vi "FTW-HTTPClient-AddHeaders.vi"(0 "HTTP Client":refnum<class "FTW-HTTPClient.lvclass">, 5 "Headers":T1[](array[typedef]), 11 "error in":errorcluster) -> (4 "HTTP Client out":refnum<class "FTW-HTTPClient.lvclass">, 15 "error out":errorcluster)   [LabVIEW 2012, in "FTW-HTTPClient.lvclass"]
uses:
  FTW-HTTPClient.lvclass
  Collection/FTW-Collection-KeyValuePair.ctl
  FTW-HTTPClient.lvclass/FTW-HTTPClient.ctl
panel:
  # "Inputs"
  # "Outputs"
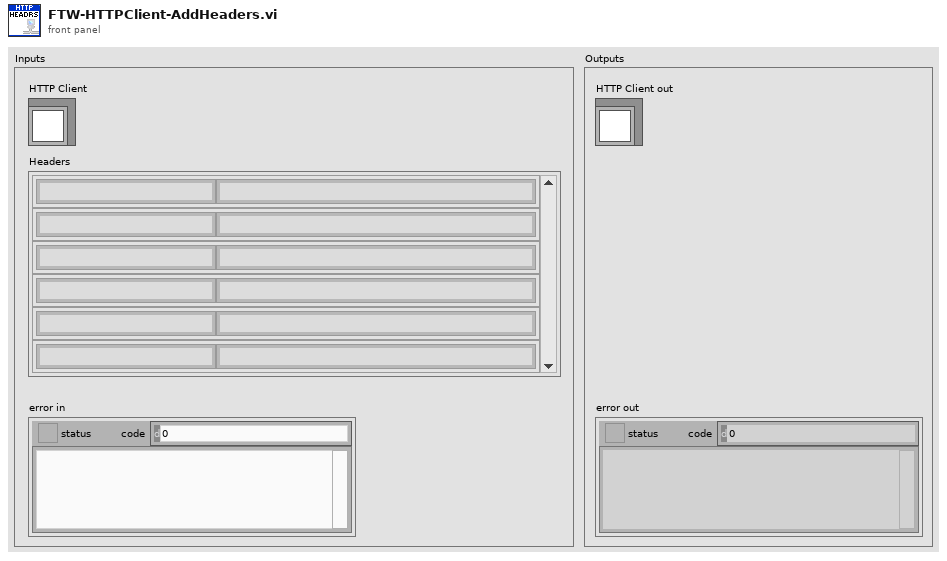
[diagram p1: front panel]
types:
  T1 = typedef "FTW-Collection-KeyValuePair.ctl" = cluster{"Key":string, "Value":string}
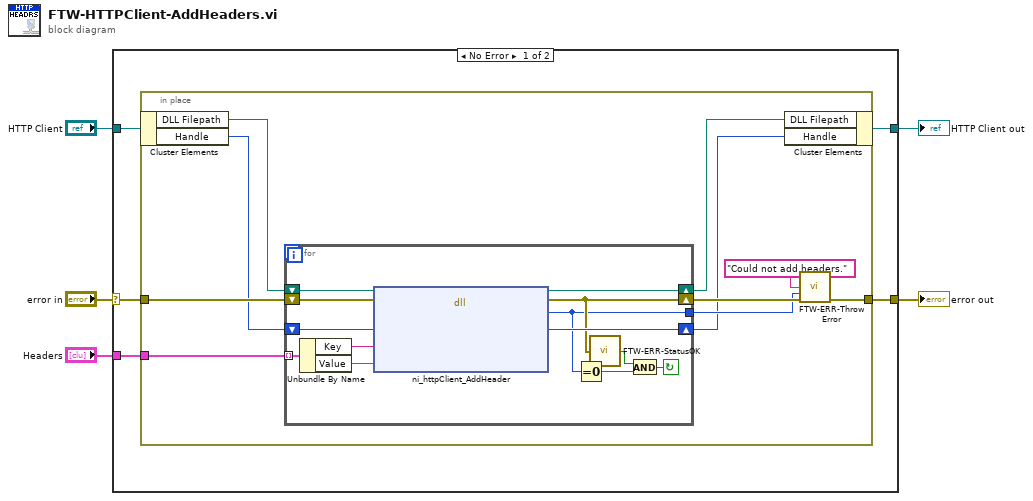
[diagram p0: block diagram]
diagram:
  n1 = case shown="No Error" "error in" {
    selector: "error in" -> [w8 w35]
    tunnel: [w7 w35] -> w5
    tunnel: "HTTP Client" -> [w10 w34]
    tunnel: [w9 w34] -> w3
    tunnel: "Headers" -> [w6 _]
    frame No Error {
      n2 = in-place {
        in-place-border: w8 -> [w16]
        in-place-border: [w19] -> w7
        in-place-border: w6 -> [w11]
        n3 = in-place-cluster #1(w10) -> ("DLL Filepath"=w18:path, "Handle"=w13:u32)
        n4 = for {
          tunnel: [w27] -> w14
          shift-right: [w32] -> w17
          shift-left: w18 -> [w33]
          shift-right: [w29] -> w12
          shift-left: w13 -> [w30]
          shift-right: [w28] -> w15
          shift-left: w16 -> [w31]
          tunnel: w11 -> [w23] mode=indexing
          stop <- w24 continue-if-true
          n5 = Unbundle By Name(w23) -> ("Key"=w22:string, "Value"=w21:string)
          n6 = dll-call lib="?" fn="ni_httpClient_AddHeader"(path in=w33, error in=w31, "Handle"=w30, "Header"=w22, "Value"=w21) -> (path out=w32:path, error out=w28:errorcluster, "Return"=w27:i32, "Handle"=w29:u32)  [unwired: 3 in]
          n7 = Equal To 0?(x=w27) -> (x = 0?=w25:bool)
          n8 = call "FTW-ERR-StatusOK.vi"("error to check"=w28) -> ("Status OK?"=w26:bool)
          n9 = And(x=w26, y=w25) -> (x .and. y?=w24:bool)
        }
        n10 = in-place-cluster #1("DLL Filepath"=w17, "Handle"=w12) -> (w9:refnum<class "FTW-HTTPClient.lvclass">)
        n11 = call "FTW-ERR-ThrowError.vi"("Error Message"="Could not add headers.", "Error Code"=w14, "error in"=w15) -> ("error out"=w19:errorcluster)  [unwired: 12 in]
      }
    }
    frame Error {
    }
  }
  "error out" <- w5
  "HTTP Client out" <- w3
